vi "PV ActiveLine - KeyLock.vi"(7 "W/R":bool, 8 "Fehler (Eingang)":errorcluster, 9 "Lock":u16(ring) items=["unlock", "lock"], 11 "Referenz in":refnum<visa-resource-name>) -> (0 "Cluster (Ausgang)":errorcluster, 1 "Read Status":u16(ring) items=["Read Failed", "Read Ok"], 2 "Status":u16(ring) items=["Unlocked", "Locked"], 3 "Referenz out":refnum<visa-resource-name>)   [LabVIEW 2013, in "PV ActiveLine.lvlib"]
doc: "LOC - Keylock\n\nTransmit: LOC [,a]\nReceive: a\n\nKeylock,\na =\n0 –> Off (default)\n1 –> On"
uses:
  <instrlib>/PV ActiveLine/PV ActiveLine.lvlib
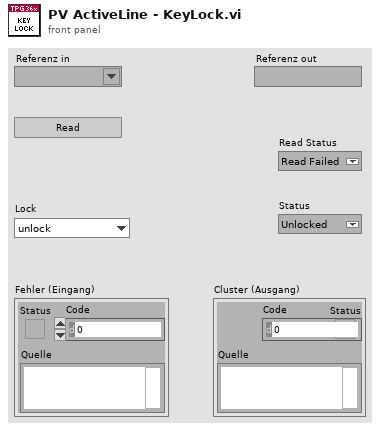
[diagram p1: front panel]
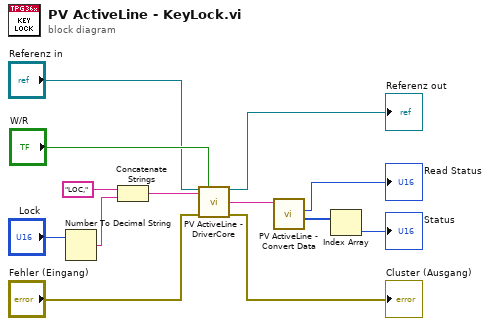
[diagram p0: block diagram]
diagram:
  n1 = Number To Decimal String(number="Lock") -> (decimal integer string=w9:string)  [unwired: 1 in]
  n2 = Concatenate Strings("LOC,", w9) -> (w11:string)
  n3 = call <instrlib>:"PV ActiveLine - DriverCore.vi"("Referenz in"="Referenz in", "Write/Read"="W/R", "Command"=w11, "Fehler (Eingang)"="Fehler (Eingang)") -> ("Referenz out"=→"Referenz out":refnum<visa-resource-name>, "String Out"=w4:string, "Cluster (Ausgang)"=→"Cluster (Ausgang)":errorcluster)  [unwired: 9 in]
  n4 = call <instrlib>:"PV ActiveLine - Convert Data.vi"("String in"=w4) -> ("Integer Out"=w2:i32[], "Read Status"=→"Read Status":u16)  [unwired: 7 in, 2 out]
  n5 = Index Array(array=w2) -> (element=→"Status":i32)  [unwired: 1 in]
